vi "SE_HV200.SetChannelsOFF.vi"(0 "i ref in":refnum<vi>, 2 "Channel":i32, 4 "Time out":i32, 5 "error in (no error)":errorcluster) -> (14 "i ref out":refnum<vi>, 16 "timed out":bool, 19 "error out":errorcluster)   [LabVIEW 2014, in "SE_HV200.lvlib"]
doc: "Sets the Voltage at the Device. but first one should increase the current to set the voltage else the Voltage might not be set"
uses:
  SE_HV200.lvlib
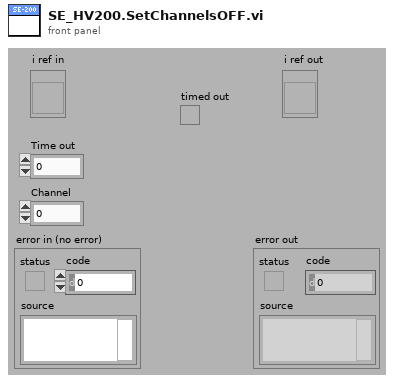
[diagram p1: front panel]
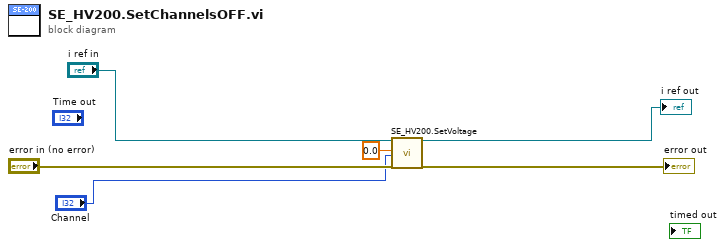
[diagram p0: block diagram]
diagram:
  n1 = call "SE_HV200.SetVoltage.vi"("i ref in"="i ref in", "Set Voltage"=0.0, "Channel"="Channel", "error in (no error)"="error in (no error)") -> ("i ref out"=→"i ref out":refnum<vi>, "error out"=→"error out":errorcluster)  [unwired: 13 in, 1 out]
